vi "transform_point.vi"(10 "Transformation":sgl[][](array[numeric]), 11 "3D Point":T1) -> (3 "output cluster":T1)   [LabVIEW 2020, in "3DPC_SurfacePlot.xctl"]
uses:
  <vilib>/Native 3D Graph/xcontrol/3DPC_SurfacePlot.xctl
  <vilib>/Utility/miscctls.llb/LV3DPointTypeDef.ctl
  <vilib>/Analysis/baseanly.llb/A x Vector.vi
  <vilib>/Analysis/NI_AALBase.lvlib
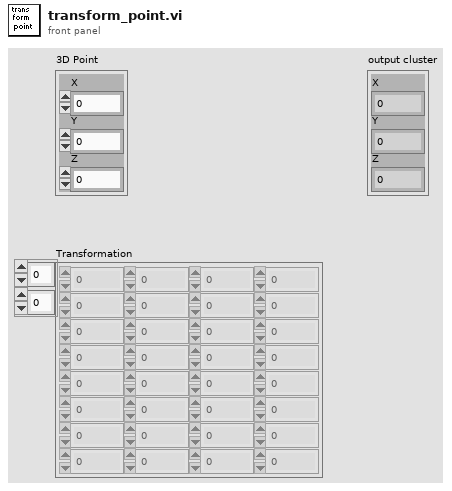
[diagram p1: front panel]
types:
  T1 = typedef "LV3DPointTypeDef.ctl" = cluster{"X":sgl, "Y":sgl, "Z":sgl}
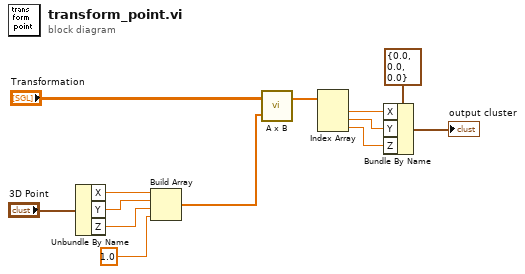
[diagram p0: block diagram]
diagram:
  n1 = Unbundle By Name("3D Point") -> ("X"=w11:sgl, "Y"=w9:sgl, "Z"=w8:sgl)
  n2 = Build Array(w11, w9, w8, sgl 1.0 ("element")) -> (w7:sgl[])
  n3 = call-poly <vilib>:"A x B.vi"("Vector"=w7, "A"="Transformation") -> ("A x Vector"=w5:dbl[])  [unwired: 1 out]
  n4 = Index Array(array=w5) -> (element #1=w4:dbl, element #2=w3:dbl, element #3=w2:dbl)  [unwired: 3 in]
  n5 = Bundle By Name(cluster=T1 {"X"=0.0, "Y"=0.0, "Z"=0.0} ("3D Point"), "X"=w4, "Y"=w3, "Z"=w2) -> (→"output cluster":T1)
